vi "Generate Legend Text.vi"(8 "Last Text":T1, 9 "Gap":i32, 11 "Width":u32) -> (0 "New Text":T1)   [LabVIEW 2016, in "CML UI.lvlib" / "Circular Cue Helper.lvlib"]
doc: "This VI generates Legend Text of pie chart."
uses:
  Circular Cue Helper.lvlib
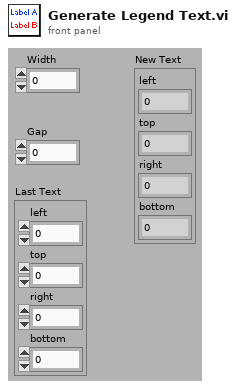
[diagram p1: front panel]
types:
  T1 = cluster{"left":i16, "top":i16, "right":i16, "bottom":i16}
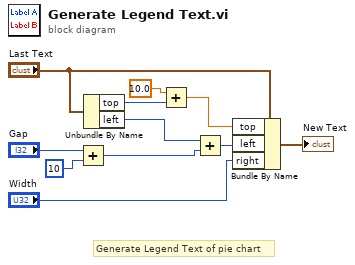
[diagram p0: block diagram]
diagram:
  # "Generate Legend Text of pie chart"
  n1 = Add(x="Gap", y=10) -> (x+y=w1:i32)
  n2 = Unbundle By Name("Last Text") -> ("top"=w10:i16, "left"=w4:i16)
  n3 = Add(x=10.0 ("y"), y=w10) -> (x+y=w11:dbl)
  n4 = Add(x=w4, y=w1) -> (x+y=w5:i32)
  n5 = Bundle By Name(cluster="Last Text", "top"=w11, "left"=w5, "right"="Width") -> (→"New Text":T1)
